vi "channel.search.vi"(8 "error in":errorcluster, 11 "Client in":refnum<class "Client.lvclass">) -> (0 "error out":errorcluster, 3 "Client out":refnum<class "Client.lvclass">)   [LabVIEW 2020, in "Client.lvclass"]
doc: "Searches for channels matching an optional data source, name substring, and data type, and returns a handle list of matches."
uses:
  Client.lvclass
  client.lvlib
panel:
  out "out_count out":u32
  out "out_list out":i32
  in  "out_count":u32
  in  "data_type":i32
  in  "substring":string
  in  "data_source_rid":string
  in  "out_list":i32
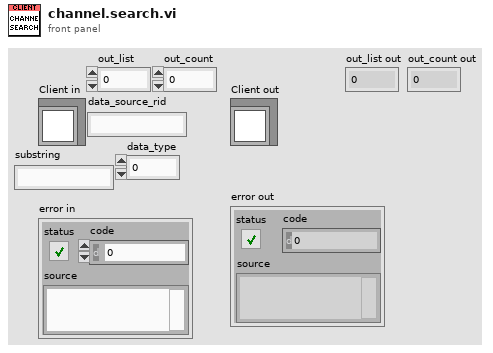
[diagram p1: front panel]
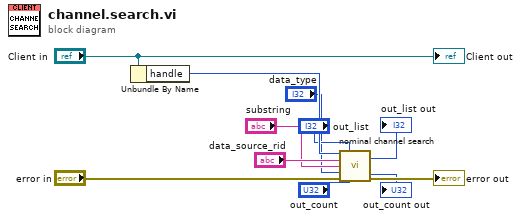
[diagram p0: block diagram]
diagram:
  n1 = Unbundle By Name("Client in") -> ("handle"=w9:i32)
  n2 = call "nominal channel search.vi"("client"=w9, "out_list"="out_list", "data_source_rid"="data_source_rid", "substring"="substring", "data_type"="data_type", "error in (no error)"="error in", "out_count"="out_count") -> ("out_list out"=→"out_list out":i32, "out_count out"=→"out_count out":u32, "error out"=→"error out":errorcluster)  [unwired: 5 in, 1 out]
  "Client out" <- "Client in"
